vi "flush.vi"(8 "Error in":errorcluster, 11 "VISA name in":refnum<visa-resource-name>) -> (0 "Error out":errorcluster, 3 "VISA name out":refnum<visa-resource-name>)   [LabVIEW 2012]
panel:
  out "文字列":string
  out "i":i32
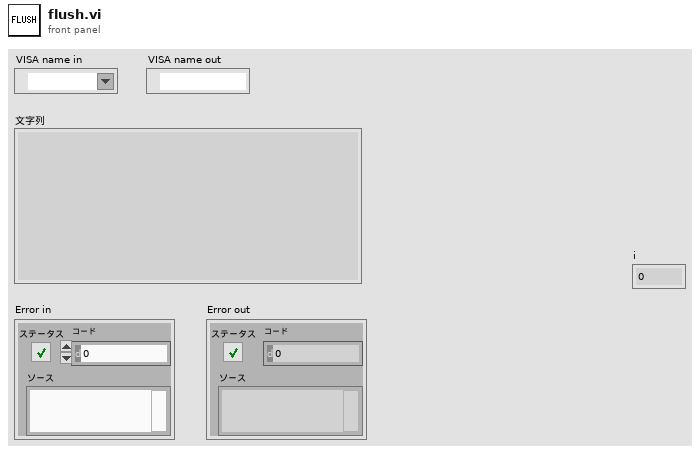
[diagram p1: front panel]
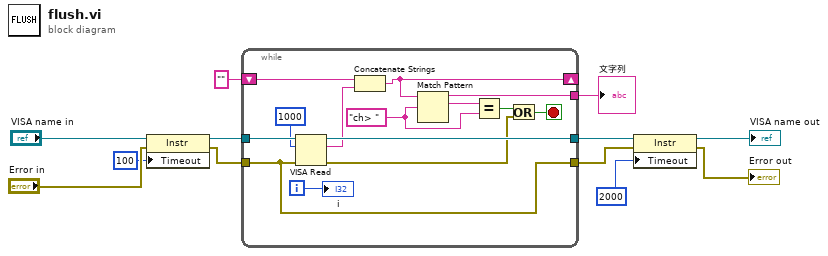
[diagram p0: block diagram]
diagram:
  n1 = property class="Instr"(reference="VISA name in", error in="Error in", "Timeout"=u32 100 ("General Settings:Timeout Value")) -> (reference out=w10:refnum<visa-resource-name>, error out=w8:errorcluster)
  n2 = while {
    shift-right: [w21] -> _
    shift-left: "" -> [w22]
    tunnel: [w20] -> w11
    tunnel: w10 -> [w26]
    tunnel: [w24] -> w5
    tunnel: w8 -> [w13]
    tunnel: [w13] -> w3
    i -> [w17]
    stop <- w16 stop-if-true
    w18 = "ch> " ("正規表現")
    n3 = VISA Read(VISA resource name=w26, byte count=u32 1000 ("バイトカウント"), error in (no error)=w13) -> (VISA resource name out=w24:refnum<visa-resource-name>, read buffer=w23:string, error out=w14:errorcluster)  [unwired: 1 out]
    n4 = Concatenate Strings(w22, w23) -> (w21:string)
    n5 = Match Pattern(string=w21, regular expression=w18) -> (before substring=w20:string, match substring=w19:string)  [unwired: 1 in, 2 out]
    n6 = Equal?(x=w19, y=w18) -> (x = y?=w15:bool)
    n7 = Or(x=w15, y=w14) -> (x .or. y?=w16:bool)
    "i" <- w17
  }
  "文字列" <- w11
  n8 = property class="Instr"(reference=w5, error in=w3, "Timeout"=u32 2000 ("General Settings:Timeout Value")) -> (reference out=→"VISA name out":refnum<visa-resource-name>, error out=→"Error out":errorcluster)
